vi "box catch act.vi"(8 "error in (no error)":errorcluster, 9 "Position":T3, 11 "main-national data":T1) -> (0 "error out":errorcluster, 1 "Position out":T3, 3 "output cluster":T1)   [LabVIEW 2019]
uses:
  ctl/main data-national.ctl
  ctl/position set.ctl
  subVI/move/position cluster.ctl
  subVI/move control/move and align/V A J control/move cluster(VAJ).ctl
  ctl/servo act.ctl
panel:
  out "catch array":string[](array[string])
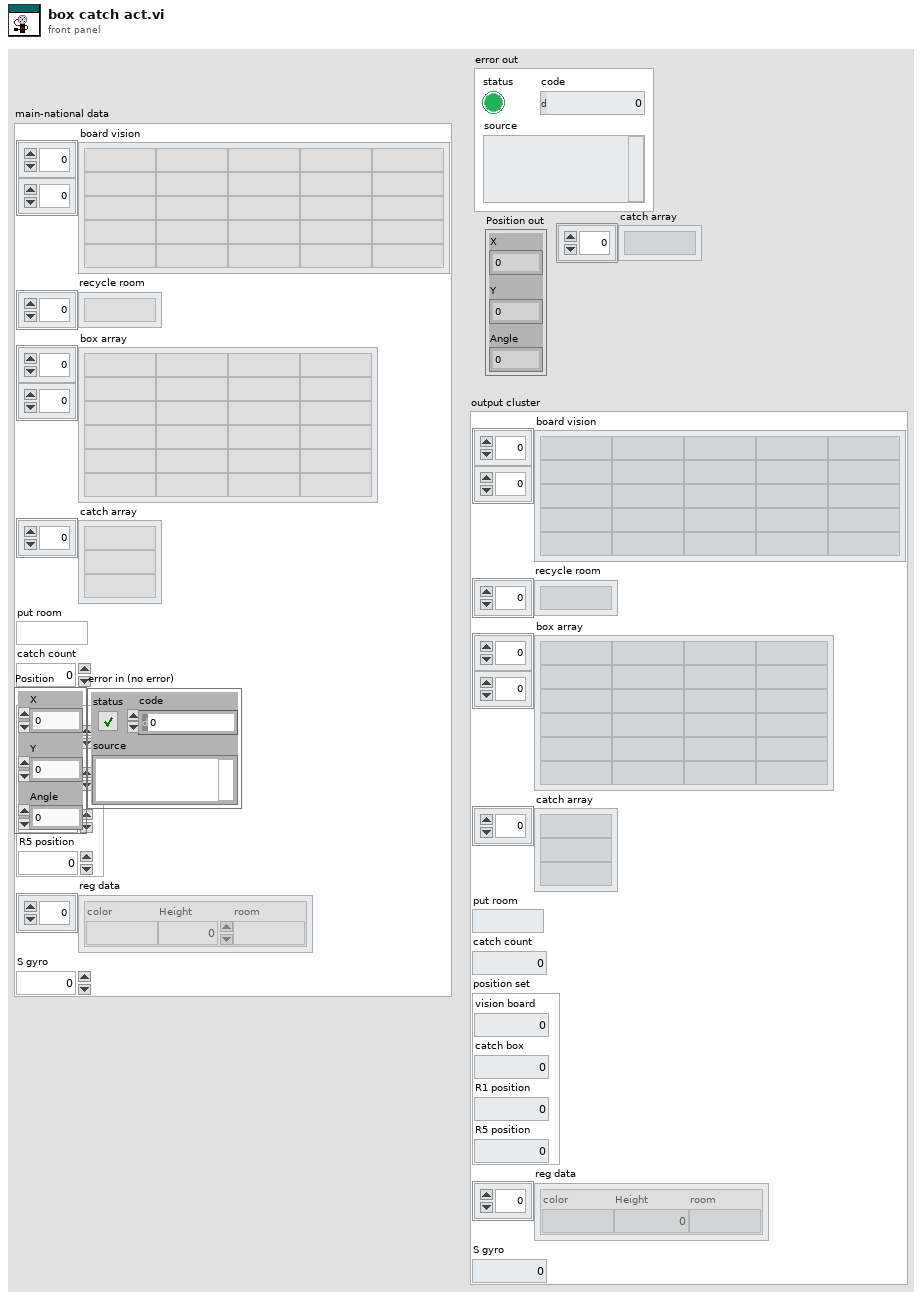
[diagram p1: front panel]
types:
  T1 = typedef "main data-national.ctl" = cluster{"board vision":string[][], "recycle room":string[], "box array":string[][], "catch array":string[], "put room":string, "catch count":dbl, "position set":T2, "reg data":cluster{"color":string, "Height":i32, "room":string}[], "S gyro":dbl}
  T2 = typedef "position set.ctl" = cluster{"vision board":dbl, "catch box":dbl, "R1 position":dbl, "R5 position":dbl}
  T3 = typedef "position cluster.ctl" = cluster{"X":dbl, "Y":dbl, "Angle":dbl}
  T4 = typedef "move cluster(VAJ).ctl" = cluster{"X":dbl, "Y":dbl, "degree":dbl, "other":string}
  T5 = typedef "servo act.ctl" = enum16{"catch", "relax", "left idle", "center", "red relax", "left reg", "right reg"}
  T6 = typedef "height.ctl" = enum16{"IDLE", "recycle pre-catch", "recycle catch", "recycle zone", "vision height", "box 1", "box 2", "box 3", "box 1 pre", "box 2 pre", "box 3 pre", "reg 1", "reg 2", "reg 1 pre", "reg 2 pre", "put 1", "put 2", "put 3"}
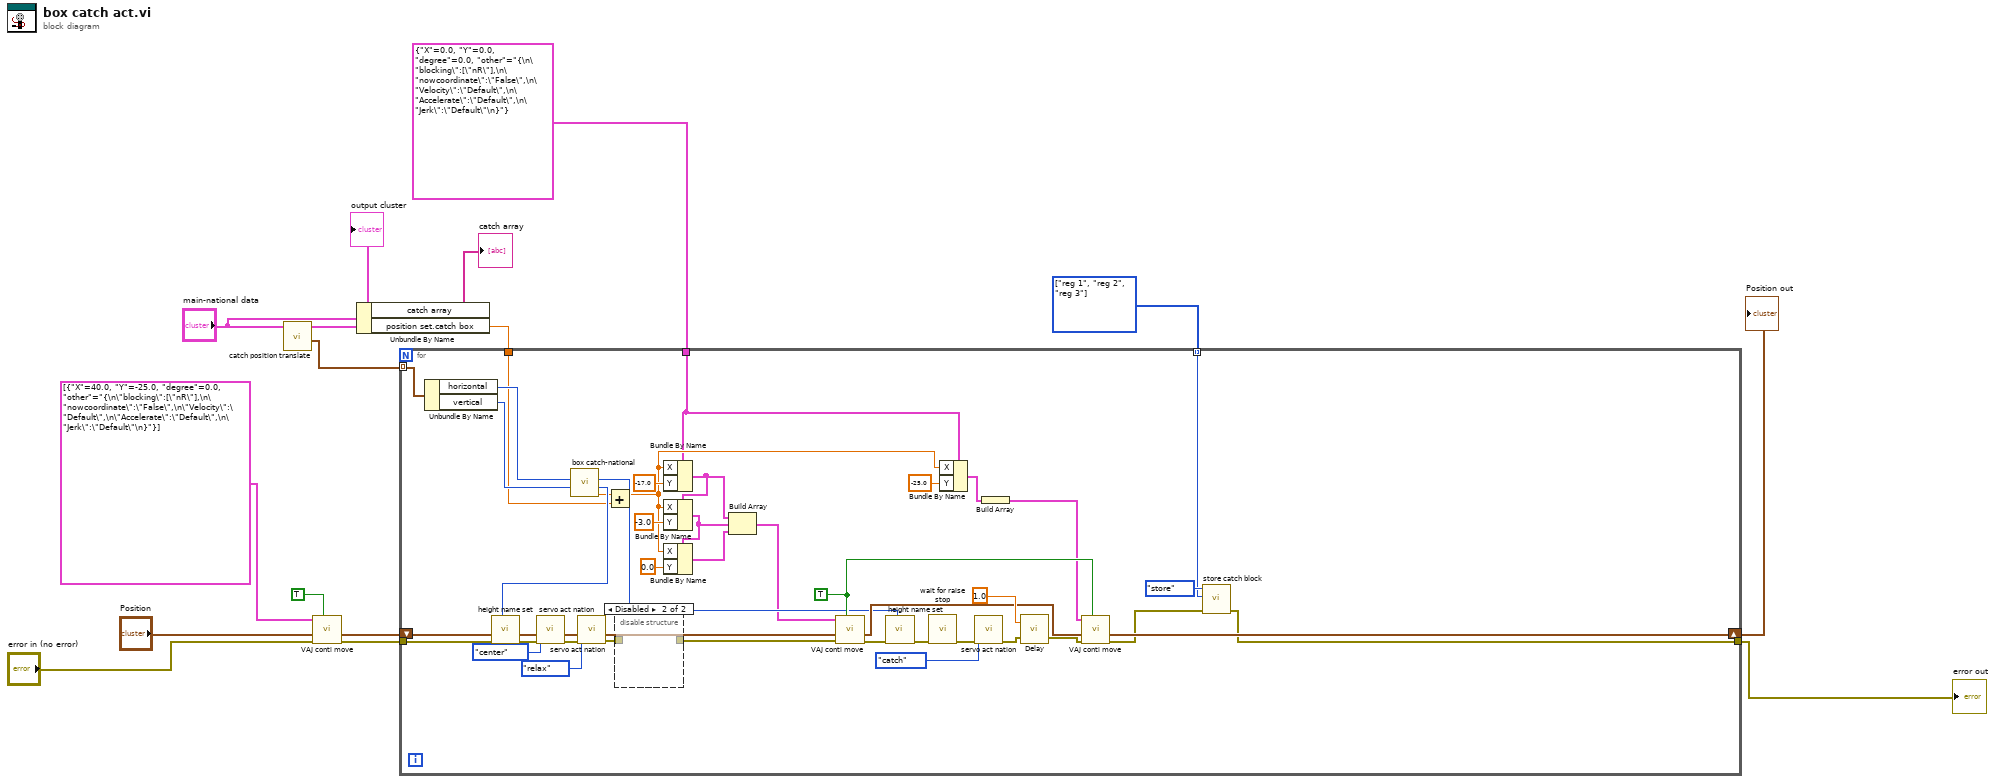
[diagram p0: block diagram]
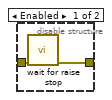
[diagram p2: hidden frame]
diagram:
  w5 = enum16{"reg 1", "reg 2", "reg 3"}[] [enum."reg 1", enum."reg 2", enum."reg 3"] items=["reg 1", "reg 2", "reg 3"] ("reg")
  n1 = call "catch position translate.vi"("main-national data"="main-national data") -> ("output position"=w15:cluster{"horizontal":i32, "vertical":i32}[], "output cluster"=→"output cluster":T1)  [unwired: 9 in]
  n2 = call "VAJ conti move.vi"("move?"=TRUE ("enable"), "error in (no error)"="error in (no error)", "Position in"="Position", "move in"=T4[] [{"X"=40.0, "Y"=-25.0, "degree"=0.0, "other"="{\n\"blocking\":[\"nR\"],\n\"nowcoordinate\":\"False\",\n\"Velocity\":\"Default\",\n\"Accelerate\":\"Default\",\n\"Jerk\":\"Default\"\n}"}]) -> ("error out"=w11:errorcluster, "Position out"=w14:T3)  [unwired: 5 in, 1 out]
  n3 = Unbundle By Name("main-national data") -> ("catch array"=→"catch array":string[], "position set.catch box"=w3:dbl)
  n4 = for {
    tunnel: w15 -> [w56] mode=indexing
    shift-right: [w28] -> w8
    shift-left: w14 -> [w53]
    tunnel: w11 -> [w46]
    tunnel: [w26] -> w10
    tunnel: w5 -> [w24] mode=indexing
    tunnel: w3 -> [w19]
    tunnel: T4 {"X"=0.0, "Y"=0.0, "degree"=0.0, "other"="{\n\"blocking\":[\"nR\"],\n\"nowcoordinate\":\"False\",\n\"Velocity\":\"Default\",\n\"Accelerate\":\"Default\",\n\"Jerk\":\"Default\"\n}"} ("move cluster(new)") -> [w18]
    w29 = TRUE ("enable")
    n5 = Unbundle By Name(w56) -> ("horizontal"=w55:i32, "vertical"=w54:i32)
    n6 = call "box catch-national.vi"("vertical"=w54, "horizontal"=w55) -> ("box X"=w32:dbl, "pre-height"=w45:T6, "height"=w21:T6)  [unwired: 7 in]
    n7 = call "height name set.vi"("height name"=w45, "error in (no error)"=w46) -> ("error out"=w44:errorcluster)  [unwired: 9 in]
    n8 = call "servo act nation.vi"("error in"=w44, "servo act"=servo_act."center") -> ("error out"=w42:errorcluster)  [unwired: 9 in]
    n9 = call "servo act nation.vi"("error in"=w42, "servo act"=servo_act."relax") -> ("error out"=w40:errorcluster)  [unwired: 9 in]
    n10 = Add(x=w32, y=w19) -> (x+y=w20:dbl)
    n11 = disable-structure shown="Disabled" {
      disable-tunnel: w40 -> [w58 _]
      disable-tunnel: [w57 _] -> w39
      frame Enabled {
        n12 = call "wait for raise stop.vi"("Error In"=w58) -> ("Error Out"=w57:errorcluster)  [unwired: 10 in]
      }
      frame Disabled {
      }
    }
    n13 = Bundle By Name(cluster=w18, "X"=w20, "Y"=-17.0) -> (w49:T4)
    n14 = Bundle By Name(cluster=w49, "X"=w20, "Y"=-3.0) -> (w48:T4)
    n15 = Bundle By Name(cluster=w48, "X"=w20, "Y"=0.0) -> (w47:T4)
    n16 = Build Array(w49, w48, w47) -> (w17:T4[])
    n17 = call "VAJ conti move.vi"("move?"=w29, "error in (no error)"=w39, "Position in"=w53, "move in"=w17) -> ("error out"=w22:errorcluster, "Position out"=w33:T3)  [unwired: 5 in, 1 out]
    n18 = call "height name set.vi"("height name"=w21, "error in (no error)"=w22) -> ("error out"=w23:errorcluster)  [unwired: 9 in]
    n19 = call "wait for raise stop.vi"("Error In"=w23) -> ("Error Out"=w38:errorcluster)  [unwired: 10 in]
    n20 = Bundle By Name(cluster=w18, "X"=w20, "Y"=-25.0) -> (w30:T4)
    n21 = call "servo act nation.vi"("error in"=w38, "servo act"=servo_act."catch") -> ("error out"=w36:errorcluster)  [unwired: 9 in]
    n22 = Build Array(w30) -> (w16:T4[])
    n23 = call "Delay.vi"("error in (no error)"=w36, "Delay Time (s)"=1.0) -> ("error out"=w34:errorcluster)  [unwired: 1 in]
    n24 = call "VAJ conti move.vi"("move?"=w29, "error in (no error)"=w34, "Position in"=w33, "move in"=w16) -> ("error out"=w27:errorcluster, "Position out"=w28:T3)  [unwired: 5 in, 1 out]
    n25 = call "store catch block.vi"("error in"=w27, "reg"=w24, "store/catch"=enum16{"store", "catch out"}."store") -> ("error out"=w26:errorcluster)  [unwired: 8 in]
  }
  "error out" <- w10
  "Position out" <- w8
